vi "Format Numeric.vi"(6 "Variant in":variant, 7 "Shift Pressed?":bool, 8 "error in":errorcluster, 10 "QD Combo Box Ref":refnum<vi>, 11 "QD Launch VI Ref":refnum<vi>) -> (0 "error out":errorcluster, 4 "Variant out":variant)   [LabVIEW 2020]
doc: "Formats selected numeric controls, indicators, and/or constants selected. The format descriptor must be entered in the Quick Drop window before activating this plugin.\n\nDefault Shortcut - [N]"
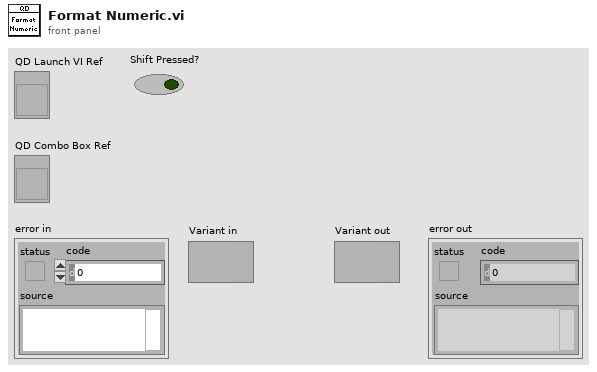
[diagram p1: front panel]
types:
  T1 = typedef "LVNumericRepresentation.ctl" = enum32{"Extended Precision", "Double Precision", "Single Precision", "Long", "Word", "Byte", "Unsigned Long", "Unsigned Word", "Unsigned Byte", "Complex Extended", "Complex Double", "Complex Single", "Quad", "Unsigned Quad", "Fixed-Point"}
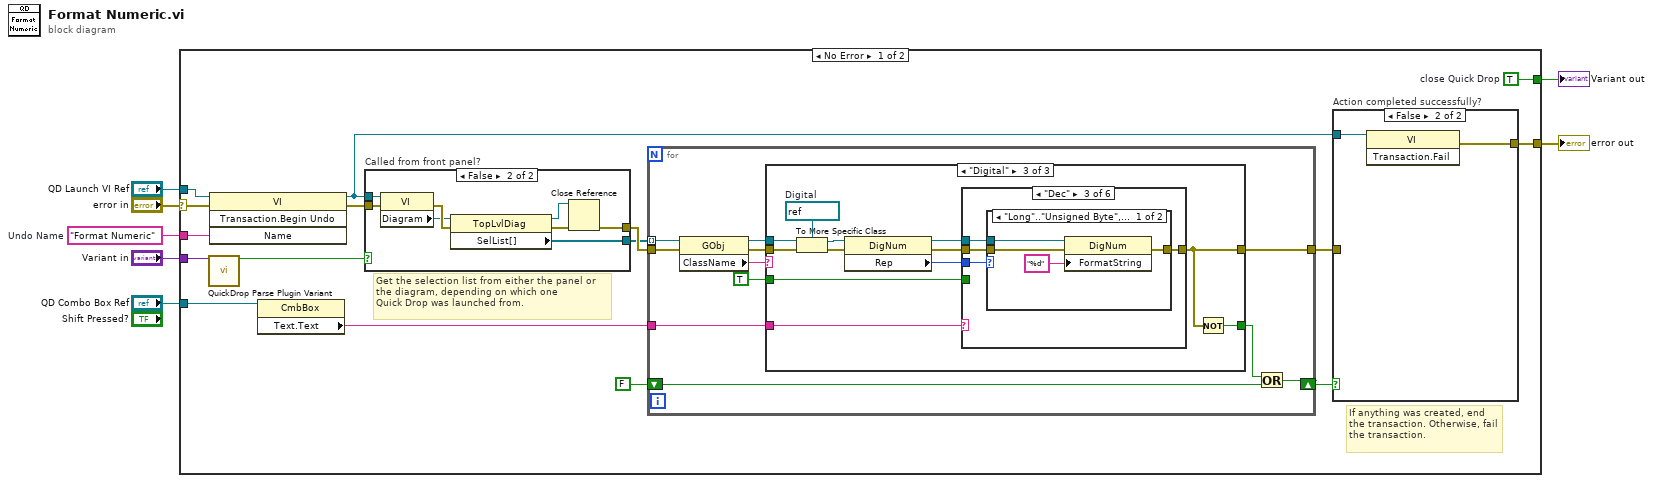
[diagram p0: block diagram]
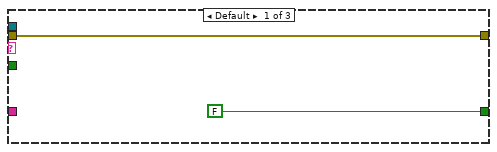
[diagram p2: hidden frame]
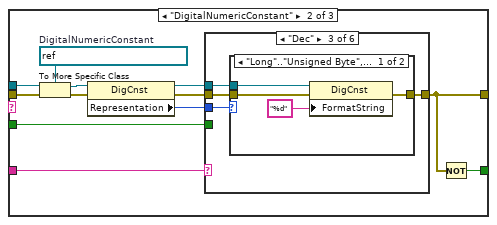
[diagram p3: hidden frame]
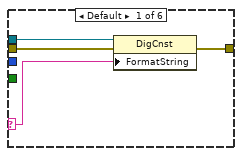
[diagram p4: hidden frame]
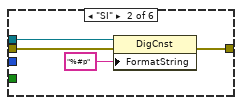
[diagram p5: hidden frame]
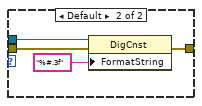
[diagram p6: hidden frame]
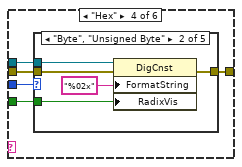
[diagram p7: hidden frame]
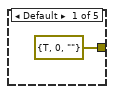
[diagram p8: hidden frame]
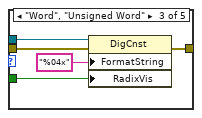
[diagram p9: hidden frame]
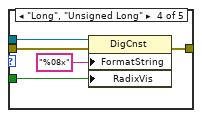
[diagram p10: hidden frame]
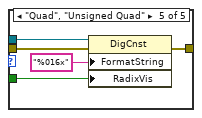
[diagram p11: hidden frame]
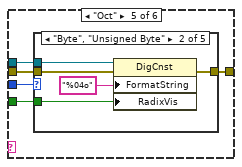
[diagram p12: hidden frame]
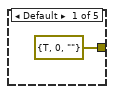
[diagram p13: hidden frame]
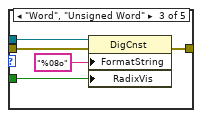
[diagram p14: hidden frame]
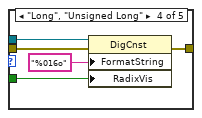
[diagram p15: hidden frame]
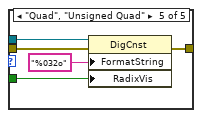
[diagram p16: hidden frame]
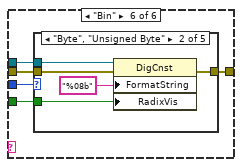
[diagram p17: hidden frame]
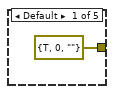
[diagram p18: hidden frame]
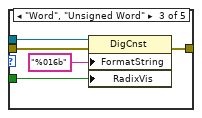
[diagram p19: hidden frame]
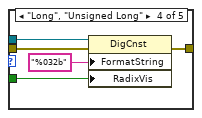
[diagram p20: hidden frame]
diagram:
  w2 = "Format Numeric"  # Undo Name
  n1 = case shown="No Error" "error in" {
    selector: "error in" -> [w22 w277]
    tunnel: [w20 w277] -> w6
    tunnel: "QD Launch VI Ref" -> [w17 _]
    tunnel: "QD Combo Box Ref" -> [w9 _]
    tunnel: "Variant in" -> [w23 _]
    tunnel: w2 -> [w16 _]
    tunnel: [w15 _] -> w1
    frame No Error {
      w15 = TRUE  # close Quick Drop
      # "Get the selection list from either the panel or\nthe diagram, depending on which one \nQuick Drop was launched from."
      # "If anything was created, end the transaction. Otherwise, fail the transaction."
      n2 = call <vilib>:"QuickDrop Parse Plugin Variant.vi"("QDKS Variant in"=w23) -> ("QD Launch VI Panel?"=w14:bool)  [unwired: 12 in, 2 out]
      n3 = invoke class="VI" method="Transaction.Begin Undo"(reference=w17, error in=w22, "Name"=w16) -> (reference out=w13:refnum<vi>, error out=w21:errorcluster)  [unwired: 1 in, 2 out]
      n4 = property class="CmbBox"(reference=w9) -> ("Text.Text"=w8:string)  [unwired: 1 in, 2 out]
      n5 = case "Called from front panel?" shown="False" w14 {
        tunnel: w21 -> [w268 w276]
        tunnel: w13 -> [w264 w272]
        tunnel: [w265 w273] -> w19
        tunnel: [w261 w269] -> w10
        frame True {
          n6 = property class="VI"(reference=w264, error in=w268) -> (error out=w267:errorcluster, "Panel"=w263:refnum<vi>)  [unwired: 1 out]
          n7 = property class="Pnl"(reference=w263, error in=w267) -> (reference out=w262:refnum<vi>, error out=w266:errorcluster, "SelList[]"=w261:refnum<vi>[])
          n8 = Close Reference(reference=w262, error in (no error)=w266) -> (error out=w265:errorcluster)
        }
        frame False {
          n9 = property class="VI"(reference=w272, error in=w276) -> (error out=w275:errorcluster, "Diagram"=w271:refnum<vi>)  [unwired: 1 out]
          n10 = property class="TopLvlDiag"(reference=w271, error in=w275) -> (reference out=w270:refnum<vi>, error out=w274:errorcluster, "SelList[]"=w269:refnum<vi>[])
          n11 = Close Reference(reference=w270, error in (no error)=w274) -> (error out=w273:errorcluster)
        }
      }
      n12 = for {
        shift-right: [w30] -> w11
        shift-left: FALSE -> [w31]
        tunnel: w10 -> [w29] mode=indexing
        tunnel: w8 -> [w27]
        tunnel: w19 -> [w34]
        tunnel: [w32] -> w18
        n13 = property class="GObj"(reference=w29, error in=w34) -> (reference out=w28:refnum<vi>, error out=w33:errorcluster, "ClassName"=w25:string)
        n14 = case shown="\"Digital\"" w25 {
          tunnel: w33 -> [w36 w48 w158]
          tunnel: w28 -> [_ w44 w154]
          tunnel: w27 -> [_ w41 w152]
          tunnel: [w36 w45 w155] -> w32
          tunnel: [FALSE w42 w153] -> w26
          tunnel: TRUE -> [_ w37 w147]
          frame Default {
          }
          frame "DigitalNumericConstant" {
            w43 = refnum<vi> refnum  # DigitalNumericConstant
            n15 = To More Specific Class(target class=w43, reference=w44, error in=w48) -> (specific class reference=w40:refnum<vi>, error out=w47:errorcluster)
            n16 = property class="DigCnst"(reference=w40, error in=w47) -> (reference out=w39:refnum<vi>, error out=w46:errorcluster, "Representation"=w38:T1)
            n17 = case shown="\"Dec\"" w41 {
              selector: w41 -> [w49 _ _ _ _ _]
              tunnel: w39 -> [w50 w54 w57 w70 w96 w122]
              tunnel: w46 -> [w52 w56 w59 w72 w98 w124]
              tunnel: [w51 w55 w60 w73 w99 w125] -> w45
              tunnel: w38 -> [_ _ w58 w71 w97 w123]
              tunnel: w37 -> [_ _ _ w69 w95 w121]
              frame Default {
                n18 = property class="DigCnst"(reference=w50, error in=w52, "FormatString"=w49) -> (error out=w51:errorcluster)  [unwired: 1 out]
              }
              frame "SI" {
                n19 = property class="DigCnst"(reference=w54, error in=w56, "FormatString"="%#p" ("Format String")) -> (error out=w55:errorcluster)  [unwired: 1 out]
              }
              frame "Dec" {
                n20 = case shown="\"Long\"..\"Unsigned Byte\", \"Quad\", \"Unsigned Quad\"" w58 {
                  tunnel: w57 -> [w62 w66]
                  tunnel: w59 -> [w64 w68]
                  tunnel: [w63 w67] -> w60
                  frame "Long".."Unsigned Byte", "Quad", "Unsigned Quad" {
                    n21 = property class="DigCnst"(reference=w62, error in=w64, "FormatString"="%d" ("Format String")) -> (error out=w63:errorcluster)  [unwired: 1 out]
                  }
                  frame Default {
                    n22 = property class="DigCnst"(reference=w66, error in=w68, "FormatString"="%#.3f" ("Format String")) -> (error out=w67:errorcluster)  [unwired: 1 out]
                  }
                }
              }
              frame "Hex" {
                n23 = case shown="\"Byte\", \"Unsigned Byte\"" w71 {
                  tunnel: w70 -> [_ w77 w82 w87 w92]
                  tunnel: w72 -> [_ w79 w84 w89 w94]
                  tunnel: [errorcluster {"status"=TRUE, "code"=0, "source"=""} ("error out") w78 w83 w88 w93] -> w73
                  tunnel: w69 -> [_ w75 w80 w85 w90]
                  frame Default {
                  }
                  frame "Byte", "Unsigned Byte" {
                    n24 = property class="DigCnst"(reference=w77, error in=w79, "FormatString"="%02x" ("Format String"), "RadixVis"=w75) -> (error out=w78:errorcluster)  [unwired: 1 out]
                  }
                  frame "Word", "Unsigned Word" {
                    n25 = property class="DigCnst"(reference=w82, error in=w84, "FormatString"="%04x" ("Format String"), "RadixVis"=w80) -> (error out=w83:errorcluster)  [unwired: 1 out]
                  }
                  frame "Long", "Unsigned Long" {
                    n26 = property class="DigCnst"(reference=w87, error in=w89, "FormatString"="%08x" ("Format String"), "RadixVis"=w85) -> (error out=w88:errorcluster)  [unwired: 1 out]
                  }
                  frame "Quad", "Unsigned Quad" {
                    n27 = property class="DigCnst"(reference=w92, error in=w94, "FormatString"="%016x" ("Format String"), "RadixVis"=w90) -> (error out=w93:errorcluster)  [unwired: 1 out]
                  }
                }
              }
              frame "Oct" {
                n28 = case shown="\"Byte\", \"Unsigned Byte\"" w97 {
                  tunnel: w96 -> [_ w103 w108 w113 w118]
                  tunnel: w98 -> [_ w105 w110 w115 w120]
                  tunnel: [errorcluster {"status"=TRUE, "code"=0, "source"=""} ("error out") w104 w109 w114 w119] -> w99
                  tunnel: w95 -> [_ w101 w106 w111 w116]
                  frame Default {
                  }
                  frame "Byte", "Unsigned Byte" {
                    n29 = property class="DigCnst"(reference=w103, error in=w105, "FormatString"="%04o" ("Format String"), "RadixVis"=w101) -> (error out=w104:errorcluster)  [unwired: 1 out]
                  }
                  frame "Word", "Unsigned Word" {
                    n30 = property class="DigCnst"(reference=w108, error in=w110, "FormatString"="%08o" ("Format String"), "RadixVis"=w106) -> (error out=w109:errorcluster)  [unwired: 1 out]
                  }
                  frame "Long", "Unsigned Long" {
                    n31 = property class="DigCnst"(reference=w113, error in=w115, "FormatString"="%016o" ("Format String"), "RadixVis"=w111) -> (error out=w114:errorcluster)  [unwired: 1 out]
                  }
                  frame "Quad", "Unsigned Quad" {
                    n32 = property class="DigCnst"(reference=w118, error in=w120, "FormatString"="%032o" ("Format String"), "RadixVis"=w116) -> (error out=w119:errorcluster)  [unwired: 1 out]
                  }
                }
              }
              frame "Bin" {
                n33 = case shown="\"Byte\", \"Unsigned Byte\"" w123 {
                  tunnel: w122 -> [_ w129 w134 w139 w144]
                  tunnel: w124 -> [_ w131 w136 w141 w146]
                  tunnel: [errorcluster {"status"=TRUE, "code"=0, "source"=""} ("error out") w130 w135 w140 w145] -> w125
                  tunnel: w121 -> [_ w127 w132 w137 w142]
                  frame Default {
                  }
                  frame "Byte", "Unsigned Byte" {
                    n34 = property class="DigCnst"(reference=w129, error in=w131, "FormatString"="%08b" ("Format String"), "RadixVis"=w127) -> (error out=w130:errorcluster)  [unwired: 1 out]
                  }
                  frame "Word", "Unsigned Word" {
                    n35 = property class="DigCnst"(reference=w134, error in=w136, "FormatString"="%016b" ("Format String"), "RadixVis"=w132) -> (error out=w135:errorcluster)  [unwired: 1 out]
                  }
                  frame "Long", "Unsigned Long" {
                    n36 = property class="DigCnst"(reference=w139, error in=w141, "FormatString"="%032b" ("Format String"), "RadixVis"=w137) -> (error out=w140:errorcluster)  [unwired: 1 out]
                  }
                  frame "Quad", "Unsigned Quad" {
                    n37 = property class="DigCnst"(reference=w144, error in=w146, "FormatString"="%064b" ("Format String"), "RadixVis"=w142) -> (error out=w145:errorcluster)  [unwired: 1 out]
                  }
                }
              }
            }
            n38 = Not(x=w45) -> (.not. x?=w42:bool)
          }
          frame "Digital" {
            w148 = refnum<vi> refnum  # Digital
            n39 = To More Specific Class(target class=w148, reference=w154, error in=w158) -> (specific class reference=w151:refnum<vi>, error out=w157:errorcluster)
            n40 = property class="DigNum"(reference=w151, error in=w157) -> (reference out=w150:refnum<vi>, error out=w156:errorcluster, "Rep"=w149:T1)
            n41 = case shown="\"Dec\"" w152 {
              selector: w152 -> [w159 _ _ _ _ _]
              tunnel: w150 -> [w160 w164 w167 w180 w206 w232]
              tunnel: w156 -> [w162 w166 w169 w182 w208 w234]
              tunnel: [w161 w165 w170 w183 w209 w235] -> w155
              tunnel: w149 -> [_ _ w168 w181 w207 w233]
              tunnel: w147 -> [_ _ _ w179 w205 w231]
              frame Default {
                n42 = property class="DigNum"(reference=w160, error in=w162, "FormatString"=w159) -> (error out=w161:errorcluster)  [unwired: 1 out]
              }
              frame "SI" {
                n43 = property class="DigNum"(reference=w164, error in=w166, "FormatString"="%#p" ("Format String")) -> (error out=w165:errorcluster)  [unwired: 1 out]
              }
              frame "Dec" {
                n44 = case shown="\"Long\"..\"Unsigned Byte\", \"Quad\", \"Unsigned Quad\"" w168 {
                  tunnel: w167 -> [w172 w176]
                  tunnel: w169 -> [w174 w178]
                  tunnel: [w173 w177] -> w170
                  frame "Long".."Unsigned Byte", "Quad", "Unsigned Quad" {
                    n45 = property class="DigNum"(reference=w172, error in=w174, "FormatString"="%d" ("Format String")) -> (error out=w173:errorcluster)  [unwired: 1 out]
                  }
                  frame Default {
                    n46 = property class="DigNum"(reference=w176, error in=w178, "FormatString"="%#.3f" ("Format String")) -> (error out=w177:errorcluster)  [unwired: 1 out]
                  }
                }
              }
              frame "Hex" {
                n47 = case shown="\"Byte\", \"Unsigned Byte\"" w181 {
                  tunnel: w180 -> [_ w187 w192 w197 w202]
                  tunnel: w182 -> [_ w189 w194 w199 w204]
                  tunnel: [errorcluster {"status"=TRUE, "code"=0, "source"=""} ("error out") w188 w193 w198 w203] -> w183
                  tunnel: w179 -> [_ w185 w190 w195 w200]
                  frame Default {
                  }
                  frame "Byte", "Unsigned Byte" {
                    n48 = property class="DigNum"(reference=w187, error in=w189, "FormatString"="%02x" ("Format String"), "RadixVis"=w185) -> (error out=w188:errorcluster)  [unwired: 1 out]
                  }
                  frame "Word", "Unsigned Word" {
                    n49 = property class="DigNum"(reference=w192, error in=w194, "FormatString"="%04x" ("Format String"), "RadixVis"=w190) -> (error out=w193:errorcluster)  [unwired: 1 out]
                  }
                  frame "Long", "Unsigned Long" {
                    n50 = property class="DigNum"(reference=w197, error in=w199, "FormatString"="%08x" ("Format String"), "RadixVis"=w195) -> (error out=w198:errorcluster)  [unwired: 1 out]
                  }
                  frame "Quad", "Unsigned Quad" {
                    n51 = property class="DigNum"(reference=w202, error in=w204, "FormatString"="%016x" ("Format String"), "RadixVis"=w200) -> (error out=w203:errorcluster)  [unwired: 1 out]
                  }
                }
              }
              frame "Oct" {
                n52 = case shown="\"Byte\", \"Unsigned Byte\"" w207 {
                  tunnel: w206 -> [_ w213 w218 w223 w228]
                  tunnel: w208 -> [_ w215 w220 w225 w230]
                  tunnel: [errorcluster {"status"=TRUE, "code"=0, "source"=""} ("error out") w214 w219 w224 w229] -> w209
                  tunnel: w205 -> [_ w211 w216 w221 w226]
                  frame Default {
                  }
                  frame "Byte", "Unsigned Byte" {
                    n53 = property class="DigNum"(reference=w213, error in=w215, "FormatString"="%04o" ("Format String"), "RadixVis"=w211) -> (error out=w214:errorcluster)  [unwired: 1 out]
                  }
                  frame "Word", "Unsigned Word" {
                    n54 = property class="DigNum"(reference=w218, error in=w220, "FormatString"="%08o" ("Format String"), "RadixVis"=w216) -> (error out=w219:errorcluster)  [unwired: 1 out]
                  }
                  frame "Long", "Unsigned Long" {
                    n55 = property class="DigNum"(reference=w223, error in=w225, "FormatString"="%016o" ("Format String"), "RadixVis"=w221) -> (error out=w224:errorcluster)  [unwired: 1 out]
                  }
                  frame "Quad", "Unsigned Quad" {
                    n56 = property class="DigNum"(reference=w228, error in=w230, "FormatString"="%032o" ("Format String"), "RadixVis"=w226) -> (error out=w229:errorcluster)  [unwired: 1 out]
                  }
                }
              }
              frame "Bin" {
                n57 = case shown="\"Byte\", \"Unsigned Byte\"" w233 {
                  tunnel: w232 -> [_ w239 w244 w249 w254]
                  tunnel: w234 -> [_ w241 w246 w251 w256]
                  tunnel: [errorcluster {"status"=TRUE, "code"=0, "source"=""} ("error out") w240 w245 w250 w255] -> w235
                  tunnel: w231 -> [_ w237 w242 w247 w252]
                  frame Default {
                  }
                  frame "Byte", "Unsigned Byte" {
                    n58 = property class="DigNum"(reference=w239, error in=w241, "FormatString"="%08b" ("Format String"), "RadixVis"=w237) -> (error out=w240:errorcluster)  [unwired: 1 out]
                  }
                  frame "Word", "Unsigned Word" {
                    n59 = property class="DigNum"(reference=w244, error in=w246, "FormatString"="%016b" ("Format String"), "RadixVis"=w242) -> (error out=w245:errorcluster)  [unwired: 1 out]
                  }
                  frame "Long", "Unsigned Long" {
                    n60 = property class="DigNum"(reference=w249, error in=w251, "FormatString"="%032b" ("Format String"), "RadixVis"=w247) -> (error out=w250:errorcluster)  [unwired: 1 out]
                  }
                  frame "Quad", "Unsigned Quad" {
                    n61 = property class="DigNum"(reference=w254, error in=w256, "FormatString"="%064b" ("Format String"), "RadixVis"=w252) -> (error out=w255:errorcluster)  [unwired: 1 out]
                  }
                }
              }
            }
            n62 = Not(x=w155) -> (.not. x?=w153:bool)
          }
        }
        n63 = Or(x=w26, y=w31) -> (x .or. y?=w30:bool)
      }
      n64 = case "Action completed successfully?" shown="False" w11 {
        tunnel: w13 -> [w257 w259]
        tunnel: [w258 w260] -> w20
        tunnel: w18 -> [_ _]
        frame True {
          n65 = invoke class="VI" method="Transaction.End Undo"(reference=w257) -> (error out=w258:errorcluster)  [unwired: 2 in, 2 out]
        }
        frame False {
          n66 = invoke class="VI" method="Transaction.Fail"(reference=w259) -> (error out=w260:errorcluster)  [unwired: 2 in, 2 out]
        }
      }
    }
    frame Error {
    }
  }
  "error out" <- w6
  "Variant out" <- w1
